vi "Adjust Command Voltage.vi"(1 "Command In":dbl[](array[numeric]), 2 "Offset":dbl) -> (0 "Command Out":dbl[](array[numeric]))   [LabVIEW 2009]
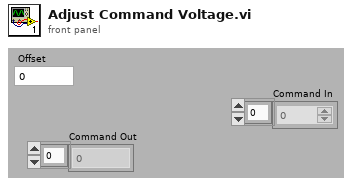
[diagram p1: front panel]
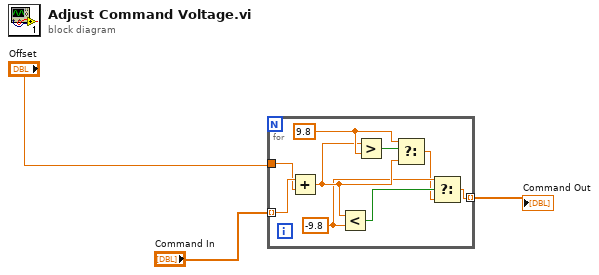
[diagram p0: block diagram]
diagram:
  n1 = for {
    tunnel: [w4] -> w1 mode=indexing
    tunnel: "Command In" -> [w12] mode=indexing
    tunnel: "Offset" -> [w11]
    w6 = -9.8 ("y")
    w8 = 9.8 ("y")
    n2 = Add(x=w12, y=w11) -> (x+y=w7:dbl)
    n3 = Less?(x=w7, y=w6) -> (x < y?=w9:bool)
    n4 = Greater?(x=w7, y=w8) -> (0:w10:bool)
    n5 = Select(t=w8, s=w10, f=w7) -> (s? t:f=w5:dbl)
    n6 = Select(t=w6, s=w9, f=w5) -> (s? t:f=w4:dbl)
  }
  "Command Out" <- w1
